vi "log_event.vi"(10 "event to log":string, 11 "log":string[](array[string])) -> (3 "log":string[](array[string]))   [LabVIEW 2016]
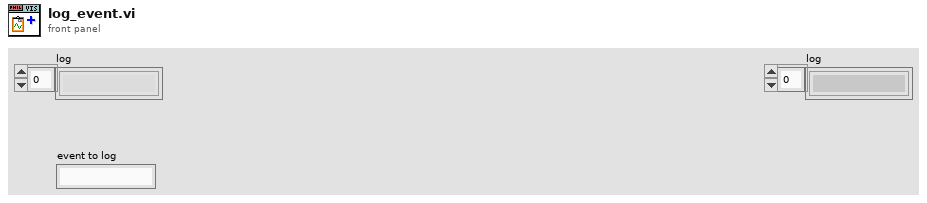
[diagram p1: front panel]
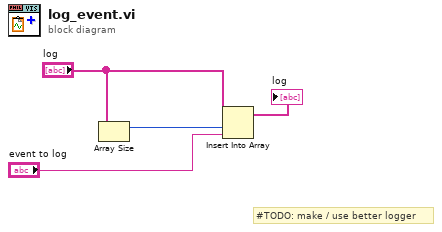
[diagram p0: block diagram]
diagram:
  # "#TODO: make / use better logger"
  n1 = Array Size(array="log") -> (size(s)=w3:i32)
  n2 = Insert Into Array(array="log", index=w3, new element="event to log") -> (→"log":string[])
